vi "Configure Clock Input Frequencies.vi"(5 "SECAM Frequency (15000 Hz)":dbl=15000.0, 6 "PAL Frequency (15000 Hz)":dbl=15000.0, 7 "NTSC Frequency (15000 Hz)":dbl=15000.0, 8 "error in (no error)":errorcluster, 9 "EXT BNC Frequency (8000 Hz)":dbl=8000.0, 10 "AES Frequency (24000 Hz)":dbl=24000.0, 11 "VISA resource name":refnum<visa-resource-name>) -> (0 "error out":errorcluster, 3 "VISA resource name out":refnum<visa-resource-name>)   [LabVIEW 2014, in "Stanford Research SR1.lvlib"]
doc: "Configures the attributes for the Clock Input Frequencies."
uses:
  Stanford Research SR1.lvlib
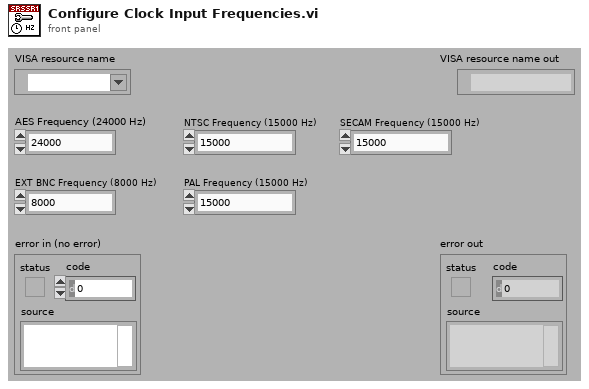
[diagram p1: front panel]
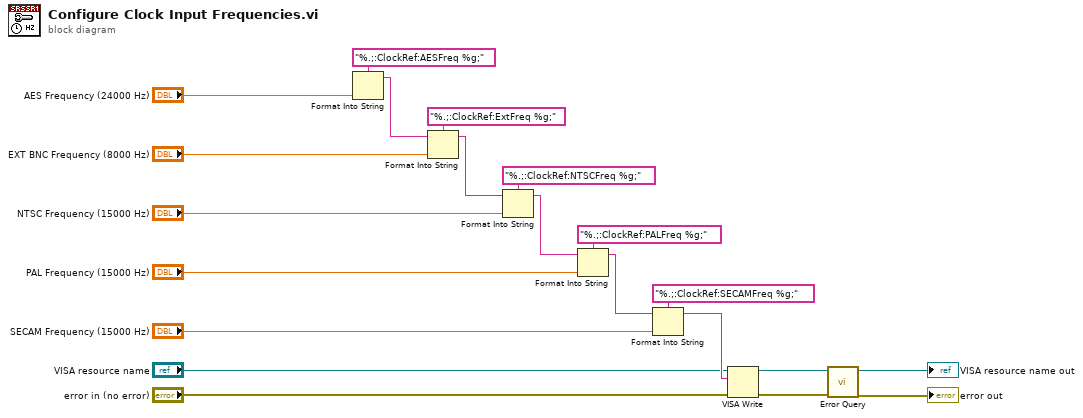
[diagram p0: block diagram]
diagram:
  n1 = Format Into String(format string="%.;:ClockRef:AESFreq %g;", "AES Frequency (24000 Hz)") -> (resulting string=w19:string)  [unwired: 2 in, 1 out]
  n2 = Format Into String(format string="%.;:ClockRef:ExtFreq %g;", initial string=w19, "EXT BNC Frequency (8000 Hz)") -> (resulting string=w16:string)  [unwired: 1 in, 1 out]
  n3 = Format Into String(format string="%.;:ClockRef:NTSCFreq %g;", initial string=w16, "NTSC Frequency (15000 Hz)") -> (resulting string=w13:string)  [unwired: 1 in, 1 out]
  n4 = Format Into String(format string="%.;:ClockRef:PALFreq %g;", initial string=w13, "PAL Frequency (15000 Hz)") -> (resulting string=w10:string)  [unwired: 1 in, 1 out]
  n5 = Format Into String(format string="%.;:ClockRef:SECAMFreq %g;", initial string=w10, "SECAM Frequency (15000 Hz)") -> (resulting string=w7:string)  [unwired: 1 in, 1 out]
  n6 = VISA Write(VISA resource name="VISA resource name", write buffer=w7, error in (no error)="error in (no error)") -> (VISA resource name out=w4:refnum<visa-resource-name>, error out=w3:errorcluster)  [unwired: 1 out]
  n7 = call "Error Query.vi"("error in (no error)"=w3, "VISA resource name"=w4) -> ("error out"=→"error out":errorcluster, "VISA resource name out"=→"VISA resource name out":refnum<visa-resource-name>)  [unwired: 6 in, 2 out]
